vi "Timer.vi"(8 "error in":errorcluster, 9 "Refresh Time":dbl=15.0, 10 "Set Time":dbl, 11 "Options":T1) -> (0 "error out":errorcluster, 2 "Elapsed?":bool, 3 "Refresh":bool)   [LabVIEW 2023, in "LTT_TeststandSteptypes.lvlib"]
uses:
  LTT_TeststandSteptypes.lvlib
  Control/TimerStates.ctl
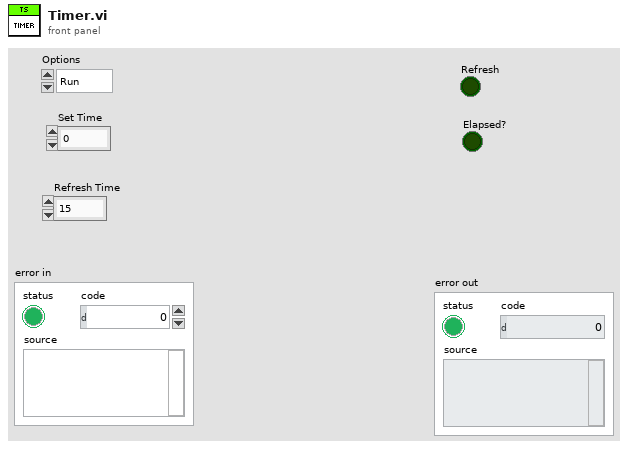
[diagram p1: front panel]
types:
  T1 = typedef "LTT_TeststandSteptypes.lvlib/TimerStates.ctl" = enum16{"Run", "Pause", "Reset"}
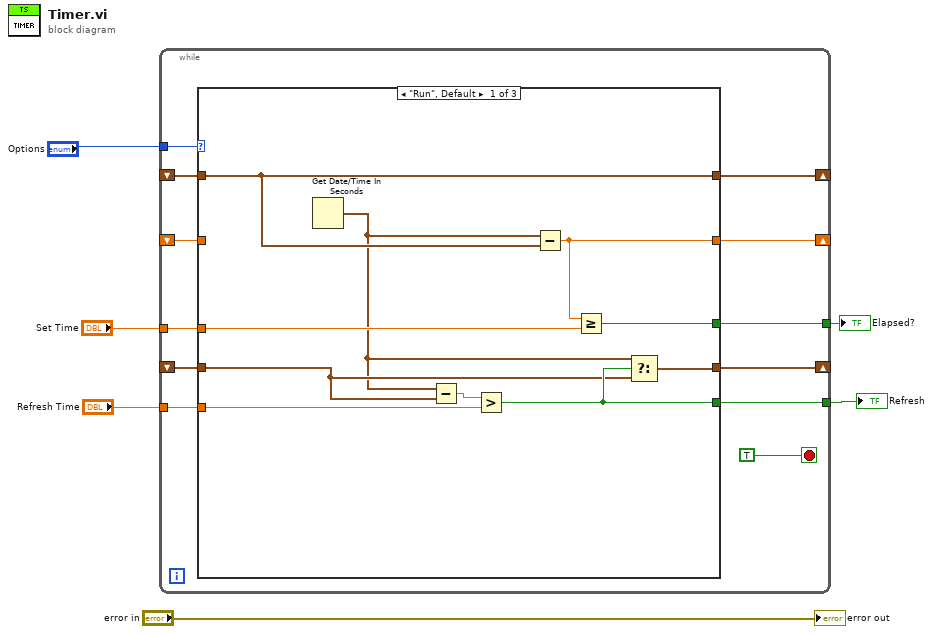
[diagram p0: block diagram]
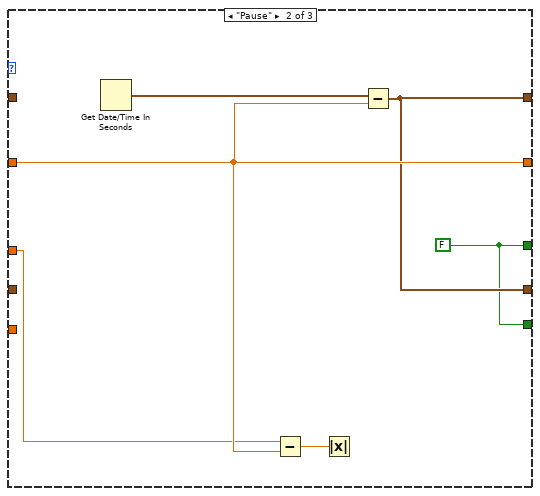
[diagram p2: hidden frame]
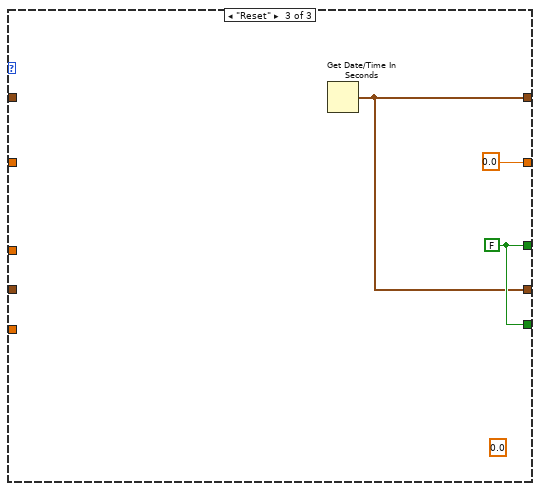
[diagram p3: hidden frame]
diagram:
  n1 = while {
    tunnel: "Options" -> [w18]
    shift-right: [w15] -> _
    shift-left: _ -> [w16]
    tunnel: "Set Time" -> [w14]
    tunnel: [w12] -> w2
    shift-right: [w13] -> _
    shift-left: _ -> [w11]
    tunnel: "Refresh Time" -> [w10]
    tunnel: [w9] -> w5
    shift-right: [w8] -> _
    shift-left: _ -> [w7]
    stop <- TRUE stop-if-true
    n2 = case shown="\"Run\", Default" w18 {
      tunnel: [w20 w33 0.0] -> w13
      tunnel: w16 -> [w28 _ _]
      tunnel: [w28 w30 w35] -> w15
      tunnel: [w27 w29 w36] -> w12
      tunnel: w14 -> [w21 w32 _]
      tunnel: w11 -> [_ w33 _]
      tunnel: w10 -> [w26 _ _]
      tunnel: [w25 w29 w36] -> w9
      tunnel: [w24 w30 w35] -> w8
      tunnel: w7 -> [w22 _ _]
      frame "Run", Default {
        n3 = Get Date/Time In Seconds() -> (seconds since 1Jan1904=w19:timestamp)
        n4 = Subtract(x=w19, y=w22) -> (x-y=w23:dbl)
        n5 = Greater?(x=w23, y=w26) -> (0:w25:bool)
        n6 = Subtract(x=w19, y=w28) -> (x-y=w20:dbl)
        n7 = Greater Or Equal?(x=w20, y=w21) -> (x >= y?=w27:bool)
        n8 = Select(t=w19, s=w25, f=w22) -> (s? t:f=w24:timestamp)
      }
      frame "Pause" {
        w29 = FALSE
        n9 = Get Date/Time In Seconds() -> (seconds since 1Jan1904=w34:timestamp)
        n10 = Subtract(x=w32, y=w33) -> (x-y=w31:dbl)
        n11 = Absolute Value(x=w31) -> ()  [unwired: 1 out]
        n12 = Subtract(x=w34, y=w33) -> (x-y=w30:timestamp)
      }
      frame "Reset" {
        (unwired) 0.0
        w36 = FALSE
        n13 = Get Date/Time In Seconds() -> (seconds since 1Jan1904=w35:timestamp)
      }
    }
  }
  "Refresh" <- w5
  "Elapsed?" <- w2
  "error out" <- "error in"
